vi "ReadTargetField.vi"(8 "error in":errorcluster) -> (0 "error out":errorcluster, 2 "Target Field (T)":dbl)   [LabVIEW 2016, in "IPS-120.lvlib" / "IPS-120-API.lvlib"]
uses:
  IPS-120-API.lvlib
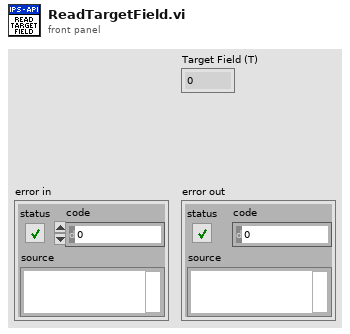
[diagram p1: front panel]
types:
  T1 = cluster{"Magnet Field":dbl, "PS Field":dbl, "Target Field":dbl, "Target Field Rate":dbl, "Voltage":dbl, "Current":dbl, "Switch":bool}
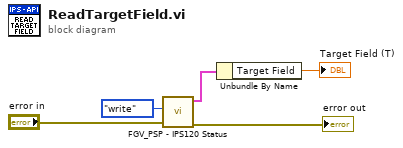
[diagram p0: block diagram]
diagram:
  n1 = call "FGV_PSP - IPS120 Status.vi"("error in"="error in", "Function"=enum16{"write", "read"}."write") -> ("error out"=→"error out":errorcluster, "status"=w2:T1)  [unwired: 4 in]
  n2 = Unbundle By Name(w2) -> ("Target Field"=→"Target Field (T)":dbl)
